vi "set_config_cluster.vi"(8 "error in (no error)":errorcluster, 10 "config cluster variant":variant, 11 "GenericPlugin in":refnum<class "StageMMS2015ASIfromScientifica.lvclass">) -> (0 "error out":errorcluster, 3 "GenericPlugin out":refnum<class "StageMMS2015ASIfromScientifica.lvclass">)   [LabVIEW 2010, in "StageMMS2015ASIfromScientifica.lvclass"]
uses:
  StageMMS2015ASIfromScientifica.lvclass
  StageMMS2015ASIfromScientifica.lvclass/StageMMS2015ASIfromScientifica.ctl
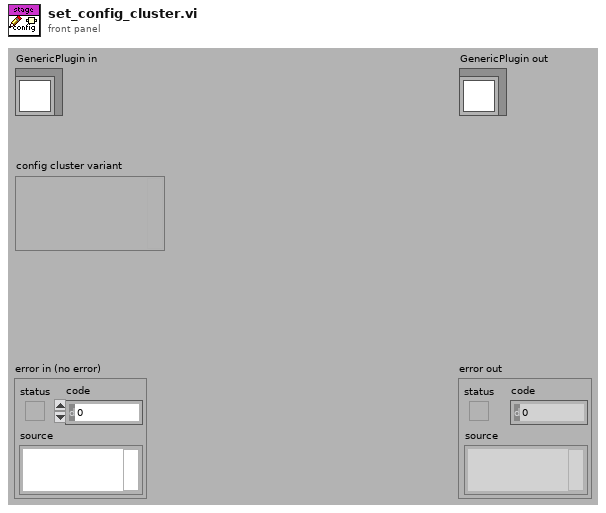
[diagram p1: front panel]
types:
  T1 = typedef "StageMMS2015ASIfromScientifica.lvclass/config_data_cluster.ctl" = cluster{"serial port name":string}
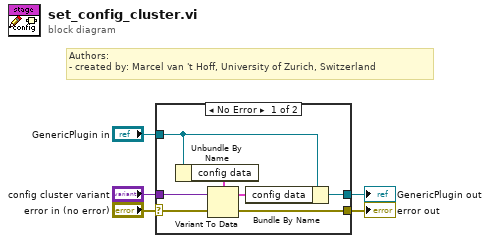
[diagram p0: block diagram]
diagram:
  # "Authors: \n- created by: Marcel van 't Hoff, University of Zurich, Switzerland"
  n1 = case shown="No Error" "error in (no error)" {
    selector: "error in (no error)" -> [w10 w13]
    tunnel: "GenericPlugin in" -> [w6 w14]
    tunnel: [w8 w13] -> w2
    tunnel: [w7 w14] -> w1
    tunnel: "config cluster variant" -> [w9 _]
    frame No Error {
      n2 = Unbundle By Name(w6) -> ("config data"=w12:T1)
      n3 = Variant To Data(error in=w10, Variant=w9, type=w12) -> (error out=w8:errorcluster, data=w11:T1)
      n4 = Bundle By Name(cluster=w6, "config data"=w11) -> (w7:refnum<class "StageMMS2015ASIfromScientifica.lvclass">)
    }
    frame Error {
    }
  }
  "error out" <- w2
  "GenericPlugin out" <- w1
